vi "ULx Read (Digital 1D Wfm NChan 1Samp).vi"(0 "task in":refnum<k24>, 9 "timeout":dbl=10.0 format="%_4g", 11 "error in":errorcluster) -> (4 "task out":refnum<k24>, 6 "data":digitalwaveform[](array[waveform]), 15 "error out":errorcluster)   [LabVIEW 2020]
doc: "Reads a waveform that contains a single sample from each channel in a task that contains one or more digital input channels."
uses:
  C:/Users/William/Documents/LV 2020 builds/LeaktestDAQ/Source-v33/ULx_LV.dll
  ULx_LV.dll
panel:
  # "channel"
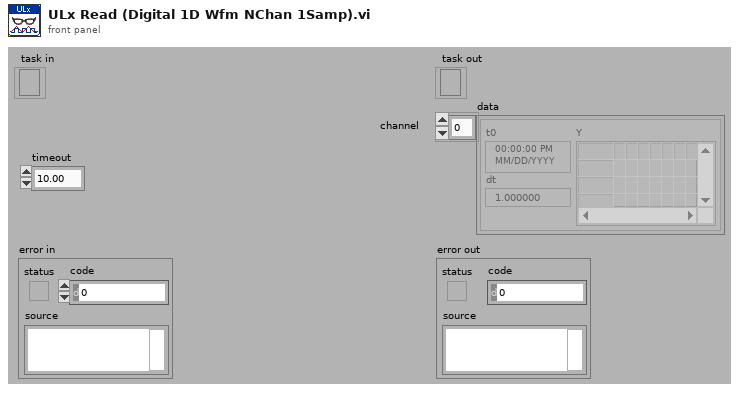
[diagram p1: front panel]
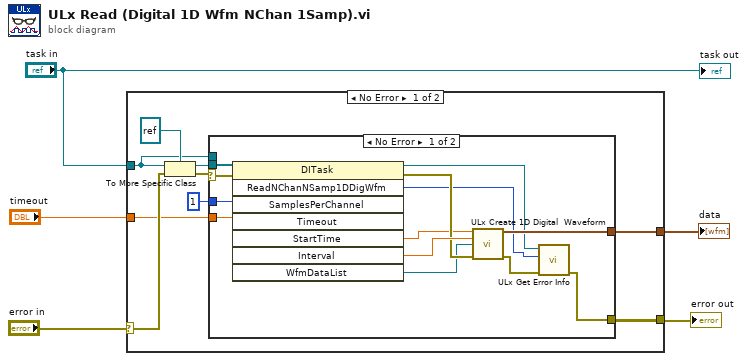
[diagram p0: block diagram]
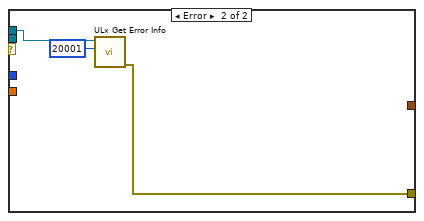
[diagram p2: hidden frame]
diagram:
  n1 = case shown="No Error" "error in" {
    selector: "error in" -> [w14 w31]
    tunnel: "task in" -> [w6 _]
    tunnel: "timeout" -> [w10 _]
    tunnel: [w9 w31] -> w3
    tunnel: [w8 _] -> w1
    frame No Error {
      n2 = To More Specific Class(target class=refnum<k24> refnum, reference=w6, error in=w14) -> (specific class reference=w11:refnum<k24>, error out=w12:errorcluster)
      n3 = case shown="No Error" w12 {
        selector: w12 -> [w26 _]
        tunnel: w11 -> [w27 _]
        tunnel: w10 -> [w25 _]
        tunnel: [w18 w28] -> w9
        tunnel: 1 ("number of samples per channel") -> [w24 _]
        tunnel: [w22 _] -> w8
        tunnel: w6 -> [_ w30]
        frame No Error {
          n4 = invoke class="DITask" method="ReadNChanNSamp1DDigWfm"(reference=w27, error in=w26, "SamplesPerChannel"=w24, "Timeout"=w25) -> (reference out=w21:refnum<k24>, error out=w20:errorcluster, "ReadNChanNSamp1DDigWfm"=w16:i32, "StartTime"=w17:dbl, "Interval"=w23:dbl, "WfmDataList"=w15:refnum<k24>)  [unwired: 4 in, 2 out]
          n5 = call "ULx Create 1D Digital  Waveform.vi"("t0"=w17, "dt"=w23, "data List"=w15, "error in"=w20) -> ("data"=w22:digitalwaveform[], "error out"=w19:errorcluster)  [unwired: 10 in]
          n6 = call "ULx Get Error Info.vi"("error in"=w19, "ErrorCode"=w16, "task in"=w21) -> ("error out"=w18:errorcluster)  [unwired: 8 in]
        }
        frame Error {
          n7 = call "ULx Get Error Info.vi"("ErrorCode"=20001, "task in"=w30) -> ("error out"=w28:errorcluster)  [unwired: 9 in]
        }
      }
    }
    frame Error {
    }
  }
  "error out" <- w3
  "data" <- w1
  "task out" <- "task in"
